vi "create client handshake initiation.vi"(10 "origin":string, 11 "websocket client in":refnum<class "websocket client.lvclass">) -> (3 "client handshake":string, 5 "accept key expected":string)   [LabVIEW 2016, in "websocket client.lvclass"]
uses:
  websocket client.lvclass
  websocket client.lvclass/websocket client.ctl
  <vilib>/wsapi/NI_WebServices.lvlib
  websocket core.lvlib
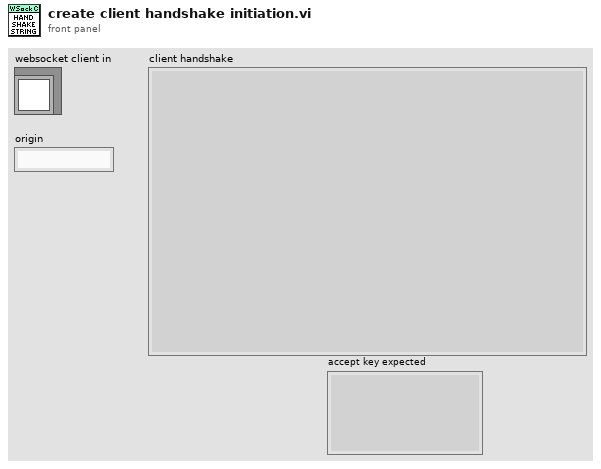
[diagram p1: front panel]
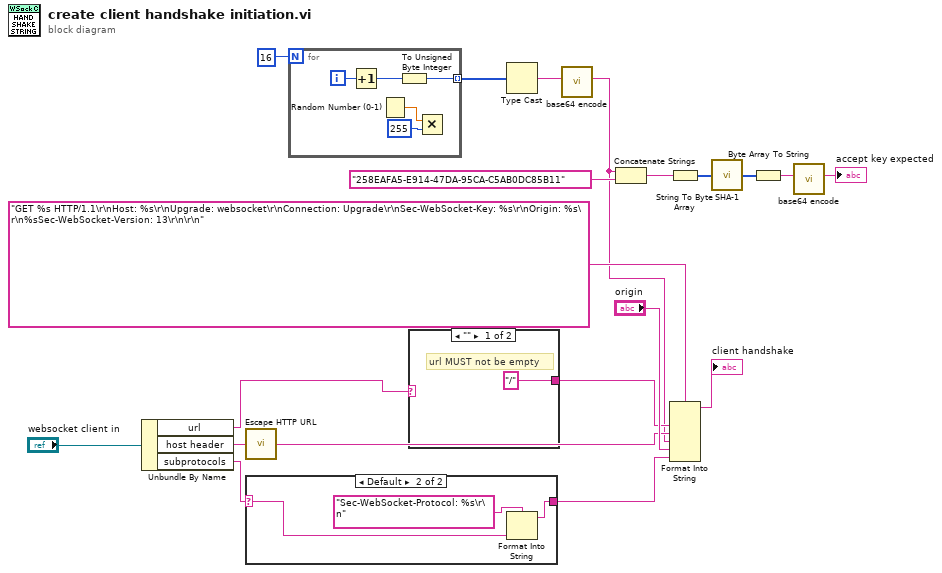
[diagram p0: block diagram]
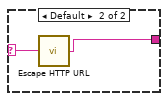
[diagram p2: hidden frame]
diagram:
  n1 = Unbundle By Name("websocket client in") -> ("url"=w1:string, "host header"=w16:string, "subprotocols"=w11:string)
  n2 = call <vilib>:"Escape HTTP URL.vi"("unescaped string in"=w16) -> ("escaped string out"=w18:string)
  n3 = case shown="Default" w11 {
    selector: w11 -> [w21 w23]
    tunnel: [w21 w22] -> w10
    frame "" {
    }
    frame Default {
      n4 = Format Into String(format string="Sec-WebSocket-Protocol: %s\r\n", w23) -> (resulting string=w22:string)  [unwired: 2 in, 1 out]
    }
  }
  n5 = for {
    N: 16 -> [_]
    tunnel: [w27] -> w12 mode=indexing
    i -> [w26]
    n6 = Increment(x=w26) -> (x+1=w25:i32)
    n7 = Random Number (0-1)() -> (number: 0 to 1=w29:dbl)
    n8 = To Unsigned Byte Integer(number=w25) -> (unsigned 8bit integer=w27:u8)
    n9 = Multiply(x=w29, y=u8 255) -> ()  [unwired: 1 out]
  }
  n10 = case shown="\"\"" w1 {
    selector: w1 -> [_ w31]
    tunnel: ["/" ("escaped string out") w32] -> w17
    frame "" {
      # "url MUST not be empty"
    }
    frame Default {
      n11 = call <vilib>:"Escape HTTP URL.vi"("unescaped string in"=w31) -> ("escaped string out"=w32:string)
    }
  }
  n12 = Type Cast(x=w12) -> (*(type *) &x=w4:string)  [unwired: 1 in]
  n13 = call "base64 encode.vi"("string in (not encoded)"=w4) -> ("string out (base64-encoded)"=w2:string)  [unwired: 10 in]
  n14 = Concatenate Strings(w2, "258EAFA5-E914-47DA-95CA-C5AB0DC85B11") -> (w8:string)
  n15 = String To Byte Array(string=w8) -> (unsigned byte array=w7:u8[])
  n16 = Format Into String(format string="GET %s HTTP/1.1\r\nHost: %s\r\nUpgrade: websocket\r\nConnection: Upgrade\r\nSec-WebSocket-Key: %s\r\nOrigin: %s\r\n%sSec-WebSocket-Version: 13\r\n\r\n", w17, w18, w2, "origin", w10) -> (resulting string=→"client handshake":string)  [unwired: 2 in, 1 out]
  n17 = call "SHA-1.vi"("Data"=w7) -> ("message-digest"=w6:u8[])
  n18 = Byte Array To String(unsigned byte array=w6) -> (string=w5:string)
  n19 = call "base64 encode.vi"("string in (not encoded)"=w5) -> ("string out (base64-encoded)"=→"accept key expected":string)  [unwired: 10 in]
